vi "GFGsectionGet.vi"(7 "GFG Refnum (use when calling from external project)":refnum<vi>, 8 "error in (no error)":errorcluster, 11 "section name":string) -> (0 "error out":errorcluster, 3 "Array of Clusters of Variables":T2(array[cluster]))   [LabVIEW 2017, in "GFG library.lvlib"]
doc: "SciScan 1.2 160622"
uses:
  GFG library.lvlib
  <vilib>/Utility/VariantDataType/Type.ctl
  <vilib>/Utility/VariantDataType/VariantType.lvlib
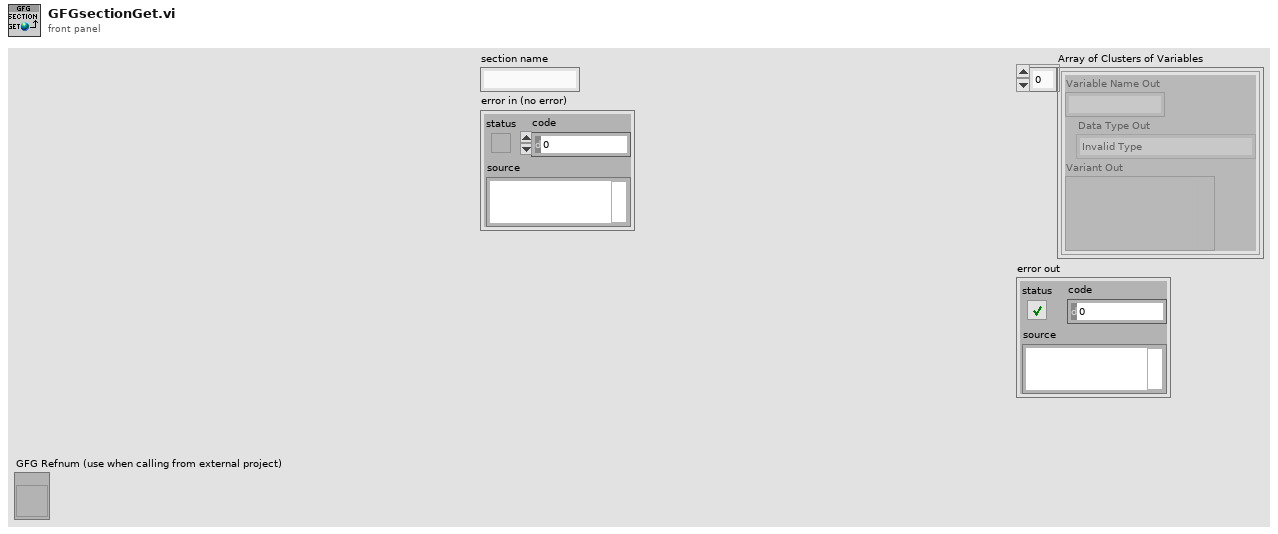
[diagram p1: front panel]
types:
  T1 = typedef "VariantType.lvlib/Type.ctl" = enum8{"Invalid Type", "Void", "I8", "I16", "I32", "I64", "U8", "U16", "U32", "U64", "Single Float", "Double Float", "Extended Float", "Single Complex", "Double Complex", "Extended Complex", "Enum U8", "Enum U16", "Enum U32", "Enum U64", "Single Float With Unit", "Double Float With Unit", "Extended Float With Unit", "Single Complex with Unit", "Double Complex with Unit", "Extended Complex with Unit", "Boolean", "String", "Path", "Picture", "Tag", "Array", "Cluster", "Variant", "LV Variant", "Waveform", "Timestamp", "Digital Waveform", "Digital Data", "ExpressData", "Refnum", "External Data", "VI", "Poly VI", "LabVIEW Class Instance", "Fixed Point"}
  T2 = cluster{"Variable Name Out":string, "Data Type Out":T1, "Variant Out":variant}[]
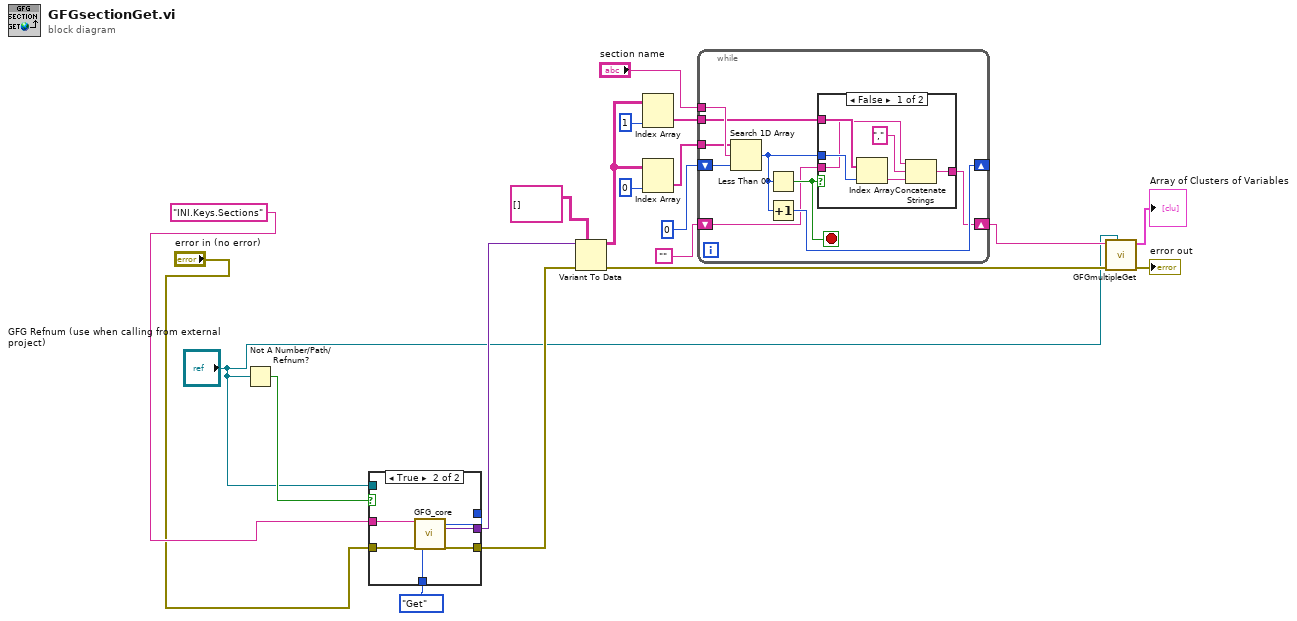
[diagram p0: block diagram]
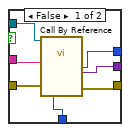
[diagram p2: hidden frame]
diagram:
  n1 = Not A Number/Path/Refnum?(number/path/refnum="GFG Refnum (use when calling from external project)") -> (NaN/Path/Refnum?=w6:bool)
  n2 = case shown="True" w6 {
    tunnel: enum16{"Init", "Set", "Get"}."Get" ("Action") -> [w22 w33]
    tunnel: "INI.Keys.Sections" ("Variable Name in") -> [w23 w32]
    tunnel: "error in (no error)" -> [w27 w31]
    tunnel: [w26 w30] -> w3
    tunnel: [w24 w29] -> _
    tunnel: [w25 w28] -> w2
    tunnel: "GFG Refnum (use when calling from external project)" -> [w21 _]
    frame False {
      n3 = call-by-ref "?"(reference=w21, "Variable Name in"=w23, "error in (no error)"=w27, "Action"=w22) -> ("Data Type Out"=w24:T1, "Variant Out"=w25:variant, "error out"=w26:errorcluster)  [unwired: 11 in, 6 out]
    }
    frame True {
      n4 = call "GFG_core.vi"("Variable Name in"=w32, "error in (no error)"=w31, "Action"=w33) -> ("Data Type Out"=w29:T1, "Variant Out"=w28:variant, "error out"=w30:errorcluster)  [unwired: 10 in, 4 out]
    }
  }
  n5 = Variant To Data(error in=w3, type=string[][] [], Variant=w2) -> (data=w15:string[][], error out=w11:errorcluster)
  n6 = Index Array(array=w15, index (col)=1 ("disabled index (col)")) -> (element=w13:string[])  [unwired: 1 in]
  n7 = Index Array(array=w15, index (col)=0 ("disabled index (col)")) -> (element=w14:string[])  [unwired: 1 in]
  n8 = while {
    tunnel: "section name" -> [w42]
    shift-right: [w39] -> _
    shift-left: 0 ("index of element") -> [w41]
    tunnel: w14 -> [w40]
    tunnel: w13 -> [w37]
    shift-right: [w34] -> w10
    shift-left: "" -> [w35]
    stop <- w38 stop-if-true
    n9 = Search 1D Array(1D array=w40, element=w42, start index (0)=w41) -> (index of element=w36:i32)
    n10 = Less Than 0?(x=w36) -> (x < 0?=w38:bool)
    n11 = Increment(x=w36) -> (x+1=w39:i32)
    n12 = case shown="False" w38 {
      tunnel: w37 -> [w46 _]
      tunnel: w36 -> [w47 _]
      tunnel: w35 -> [w44 w49]
      tunnel: [w43 w49] -> w34
      frame False {
        n13 = Index Array(array=w46, index=w47) -> (element=w45:string)
        n14 = Concatenate Strings(w44, "," ("string"), w45) -> (w43:string)
      }
      frame True {
      }
    }
  }
  n15 = call "GFGmultipleGet.vi"("GFG Refnum (use when calling from external project)"="GFG Refnum (use when calling from external project)", "error in (no error)"=w11, "comma separated\nvariable names"=w10) -> ("error out"=→"error out":errorcluster, "Array of Clusters of Variables"=→"Array of Clusters of Variables":T2)  [unwired: 7 in]
